vi "set_params.vi"(8 "error in (no error)":errorcluster caption="entrée d'erreur (pas d'erreur)", 11 "BayesianGaussianMixture.lvclass 2":refnum<class "BayesianGaussianMixture.lvclass">) -> (0 "error out":errorcluster caption="sortie d'erreur", 3 "BayesianGaussianMixture.lvclass":refnum<class "BayesianGaussianMixture.lvclass">)   [LabVIEW 2020, in "BayesianGaussianMixture.lvclass"]
uses:
  BayesianGaussianMixture.lvclass
  BayesianGaussianMixture.lvclass/BayesianGaussianMixture.ctl
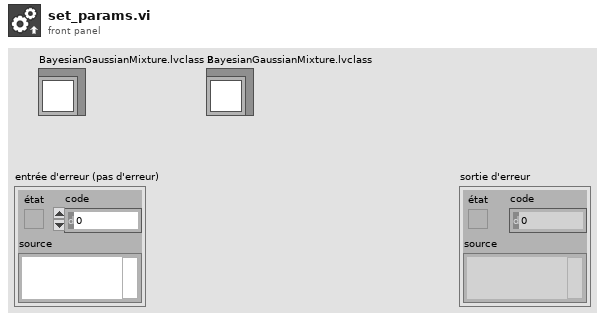
[diagram p1: front panel]
types:
  T1 = typedef "bayesian_gaussian_mixture_params.ctl" = cluster{"n_components":dbl, "covariance_type":string, "tol":dbl, "reg_covar":dbl, "max_iter":dbl, "n_init":dbl, "init_params":string, "weight_concentration_prior_type":string, "weight_concentration_prior":cluster{"weight_concentration_prior_type":string, "weight_concentration_prior_float":dbl}, "mean_precision_prior":dbl, "mean_prior":cluster{"mean_prior_type":string, "mean_prior_list":dbl[]}, "degrees_of_freedom_prior":cluster{"degrees_of_freedom_prior_type":string, "degrees_of_freedom_prior_float":dbl}, "covariance_prior":cluster{"covariance_prior_type":string, "covariance_prior_float":dbl, "covariance_prior_list":dbl[][]}, "random_state":dbl, "warm_start":bool, "verbose":dbl, "verbose_interval":dbl}
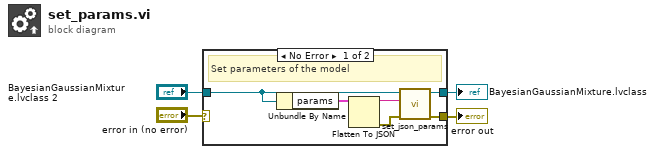
[diagram p0: block diagram]
diagram:
  n1 = case shown="No Error" "error in (no error)" {
    selector: "error in (no error)" -> [_ w12]
    tunnel: [w7 w12] -> w3
    tunnel: [w8 w11] -> w1
    tunnel: "BayesianGaussianMixture.lvclass 2" -> [w5 w11]
    frame No Error {
      # "Set parameters of the model"
      n2 = Unbundle By Name(w5) -> ("params"=w10:T1)
      n3 = Flatten To JSON(anything=w10) -> (JSON string=w9:string, 11:w6:errorcluster)  [unwired: 2 in]
      n4 = call-dynamic "set_json_params.vi"("error in (no error)"=w6, "params"=w9, "Model en entrée"=w5) -> ("error out"=w7:errorcluster, "Model en sortie"=w8:refnum<class "BayesianGaussianMixture.lvclass">)  [unwired: 7 in]
    }
    frame Error {
    }
  }
  "error out" <- w3
  "BayesianGaussianMixture.lvclass" <- w1
